vi "Fill FIFO Buffers.vi"(8 "error in (no error)":errorcluster, 11 "Refnum in":refnum<k20>) -> (0 "error out":errorcluster, 3 "Refnum out":refnum<k20>)   [LabVIEW 2014]
uses:
  <vilib>/Utility/error.llb/Error Cluster From Error Code.vi
  <vilib>/rvi/errors/niLvFpgaAdjustHostInterfaceError.vi
  <vilib>/rvi/interface/nirviMethod/nirviMethod.xnode
  <vilib>/rvi/interface/nirviReadWriteControl/nirviReadWriteControl.xnode
  <vilib>/FPGAPlugInAG/Dynamic/niLvFpga_ReadFifo_Dynamic.vi
  <vilib>/rvi/errors/niLvFpgaMergeErrorWithErrorCode.vi
  NiFpgaLv.dll
  <vilib>/rvi/interface/Simulation/niFpgaSimulationCallBeginRW.vi
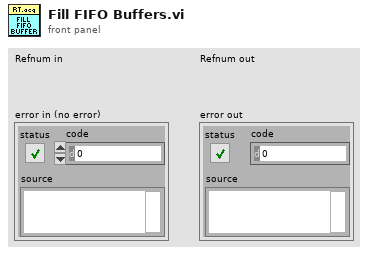
[diagram p1: front panel]
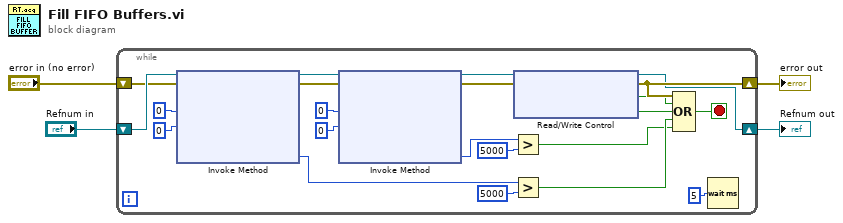
[diagram p0: block diagram]
diagram:
  n1 = while {
    shift-right: [w12] -> w3
    shift-left: "error in (no error)" -> [w25]
    shift-right: [w11] -> w4
    shift-left: "Refnum in" -> [w26]
    stop <- w6 stop-if-true
    n2 = xnode "Invoke Method"("FPGA VI Reference In"=w26, "error in"=w25, "Number of Elements"=u32 0, "Timeout (ms)"=0) -> ("FPGA VI Reference Out"=w19:refnum<k20>, "error out"=w20:errorcluster, "Elements Remaining"=w18:u32)  [unwired: 1 out]
    n3 = xnode "Invoke Method"("FPGA VI Reference In"=w19, "error in"=w20, "Number of Elements"=u32 0, "Timeout (ms)"=0) -> ("FPGA VI Reference Out"=w14:refnum<k20>, "error out"=w13:errorcluster, "Elements Remaining"=w15:u32)  [unwired: 1 out]
    n4 = Greater?(x=w15, y=u32 5000) -> (0:w7:bool)
    n5 = Greater?(x=w18, y=u32 5000) -> (0:w8:bool)
    n6 = xnode "Read/Write Control"("FPGA VI Reference In"=w14, "error in"=w13) -> ("FPGA VI Reference Out"=w11:refnum<k20>, "error out"=w12:errorcluster, "TempFIFOTimedOut?"=w10:bool, "pHFIFOTimedOut?"=w9:bool)
    n7 = Compound Arithmetic op=OR(w12, w10, w9, w8, w7) -> (w6:bool)
    n8 = Wait (ms)(milliseconds to wait=u32 5) -> ()  [unwired: 1 out]
  }
  "Refnum out" <- w4
  "error out" <- w3
